vi "wmf_set_property.vi"(7 "Auto":bool=TRUE, 8 "error in (no error)":errorcluster, 9 "Value":sgl, 10 "property name":string, 11 "camera_name":string) -> (0 "error out":errorcluster)   [LabVIEW 2024, in "Vision.lvlib"]
uses:
  Vision.lvlib
  bin/Camera.dll
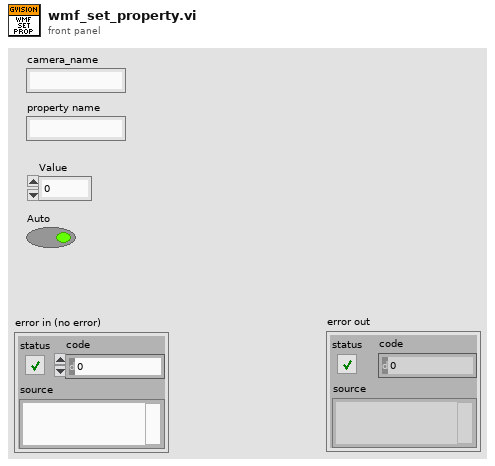
[diagram p1: front panel]
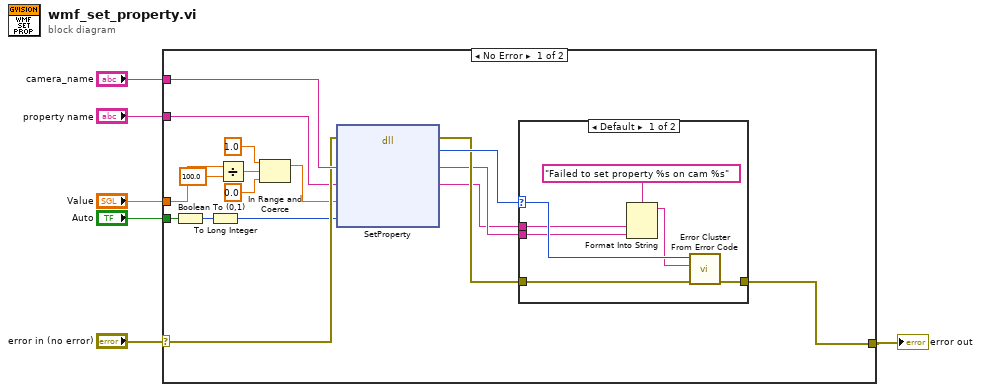
[diagram p0: block diagram]
diagram:
  n1 = case shown="No Error" "error in (no error)" {
    selector: "error in (no error)" -> [w19 w32]
    tunnel: [w21 w32] -> w4
    tunnel: "camera_name" -> [w20 _]
    tunnel: "property name" -> [w18 _]
    tunnel: "Value" -> [w12 _]
    tunnel: "Auto" -> [w15 _]
    frame No Error {
      n2 = Boolean To (0,1)(Boolean=w15) -> (0, 1=w14:i16)
      n3 = To Long Integer(number=w14) -> (32bit integer=w13:i32)
      n4 = Divide(x=w12, y=sgl 100.0) -> (x/y=w10:sgl)
      n5 = In Range and Coerce(upper limit=sgl 1.0, x=w10, lower limit=sgl 0.0) -> (coerced(x)=w7:sgl)  [unwired: 1 out]
      n6 = dll-call lib="C:/Users/cfang/Desktop/nebraska-silicon-lab/pixel-gantry-control/Gantry/Shared Components/bin/Camera.dll" fn="SetProperty"(error in=w19, "camera_name"=w20, "prop name"=w18, "val"=w7, "auto"=w13) -> (error out=w22:errorcluster, "return type"=w23:i32, "camera_name"=w17:string, "prop name"=w16:string)  [unwired: 4 in, 1 out]
      n7 = case shown="Default" w23 {
        selector: w23 -> [w28 _]
        tunnel: w22 -> [w30 w31]
        tunnel: [w29 w31] -> w21
        tunnel: w17 -> [w24 _]
        tunnel: w16 -> [w25 _]
        frame Default {
          n8 = Format Into String(format string="Failed to set property %s on cam %s" ("error message (\"\")"), w25, w24) -> (resulting string=w26:string)  [unwired: 2 in, 1 out]
          n9 = call <vilib>:"Error Cluster From Error Code.vi"("error in (no error)"=w30, "error message (\"\")"=w26, "error code (0)"=w28) -> ("error out"=w29:errorcluster)  [unwired: 6 in]
        }
        frame 0 {
        }
      }
    }
    frame Error {
    }
  }
  "error out" <- w4
